vi "Close Hardware.vi"(8 "error in (no error)":errorcluster, 11 "Instrument.FrameworkTemplate":refnum<class "Temperhum.Thorlabs.lvclass">) -> (0 "error out":errorcluster, 3 "Instrument.FrameworkTemplate out":refnum<class "Temperhum.Thorlabs.lvclass">)   [LabVIEW 2019, in "Temperhum.Thorlabs.lvclass"]
uses:
  Temperhum.Thorlabs.lvclass
  Temperhum.Thorlabs.lvclass/Temperhum.Thorlabs.ctl
  Instrument.Temperhum/Instrument.Temperhum.lvclass
  drivers/TLTSP/TLTSP.lvlib
  drivers/TLTSPB/TLTSPB.lvlib
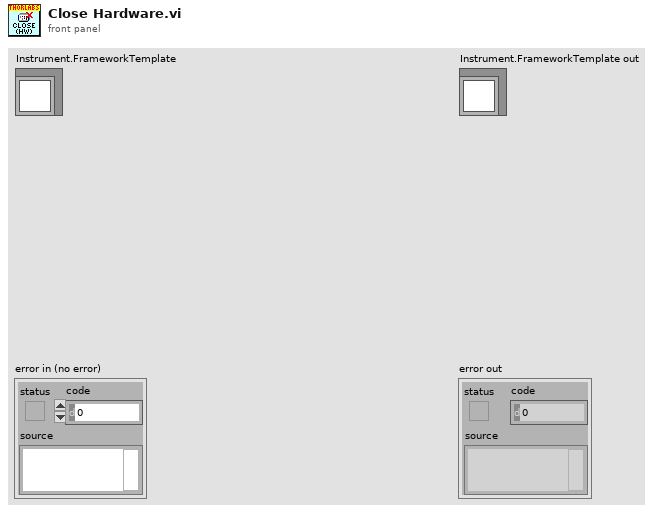
[diagram p1: front panel]
types:
  T1 = typedef "Temperhum.Thorlabs.lvclass/Thorlabs Type --enum.ctl" = enum16{"A", "B"}
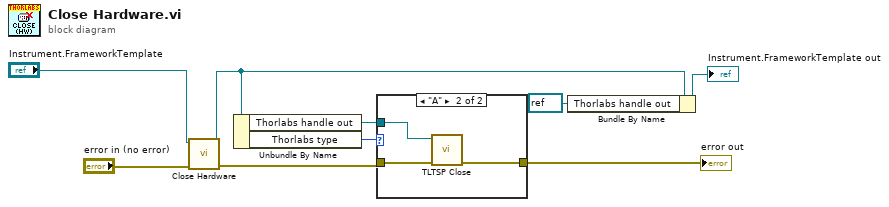
[diagram p0: block diagram]
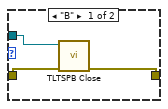
[diagram p2: hidden frame]
diagram:
  n1 = call-parent "Close Hardware.vi"("error in (no error)"="error in (no error)", "Instrument.FrameworkTemplate"="Instrument.FrameworkTemplate") -> ("error out"=w7:errorcluster, "Instrument.FrameworkTemplate out"=w3:refnum<class "Temperhum.Thorlabs.lvclass">)  [unwired: 8 in]
  n2 = Unbundle By Name(w3) -> ("Thorlabs handle out"=w1:refnum<visa-resource-name>, "Thorlabs type"=w5:T1)
  n3 = case shown="\"A\"" w5 {
    tunnel: w1 -> [w12 w13]
    tunnel: w7 -> [w11 w14]
    tunnel: [w10 w15] -> w6
    frame "B" {
      n4 = call "TLTSPB Close.vi"("error in (no error)"=w11, "instrument handle"=w12) -> ("error out"=w10:errorcluster)  [unwired: 9 in]
    }
    frame "A" {
      n5 = call "TLTSP Close.vi"("error in (no error)"=w14, "instrument handle"=w13) -> ("error out"=w15:errorcluster)  [unwired: 9 in]
    }
  }
  "error out" <- w6
  n6 = Bundle By Name(cluster=w3, "Thorlabs handle out"=refnum<visa-resource-name> refnum) -> (→"Instrument.FrameworkTemplate out":refnum<class "Temperhum.Thorlabs.lvclass">)
